vi "Automatic Teller Machine (ATM).vi"() -> ()   [LabVIEW 2016]
uses:
  Controls/State.ctl
panel:
  in  "Enter":bool
  in  "User Input":string
  in  "Right Buttons":T1
  out "Right Menu":T2
  in  "Left Buttons":T1
  out "Left Menu":T2
  in  "Card Simulator":bool
  out "ATM Messages":string
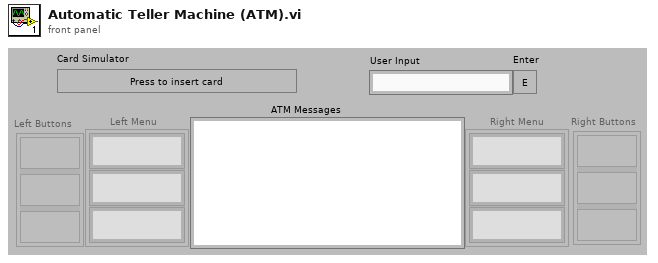
[diagram p1: front panel]
types:
  T1 = cluster{"Func Button":bool, "Func Button 2":bool, "Func Button 3":bool}
  T2 = cluster{"RFS String":string, "RFS String 2":string, "RFS String 3":string}
  T3 = typedef "State.ctl" = enum16{"Start", "Idle", "Deposit", "Withdraw", "FastCash", "None", "BalanceInquiry", "ReturnCard"}
  T4 = enum16{"CheckAccountNumber", "ReturnInfo", "Deposit", "Withdraw"}
  T5 = enum8{"Enabled", "Disabled", "Disabled and Grayed Out"}
  T6 = typedef "Account.ctl" = cluster{"Number":string, "FirstName":string, "LastName":string, "Balance":string}
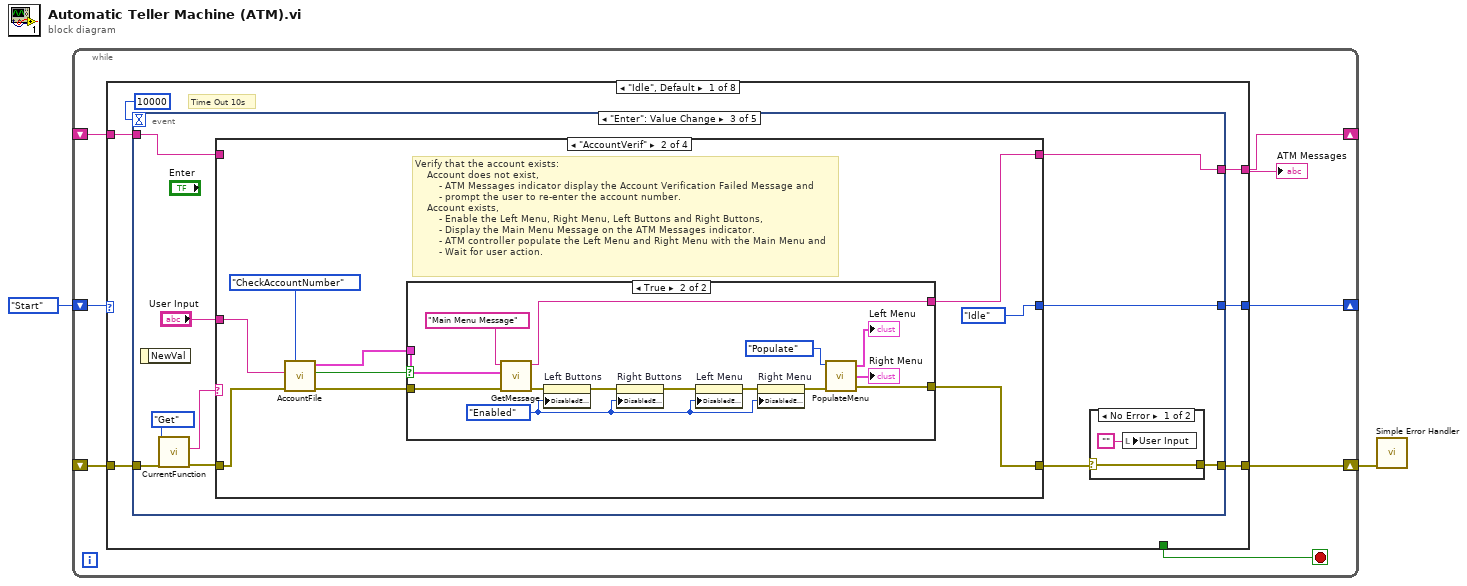
[diagram p0: block diagram]
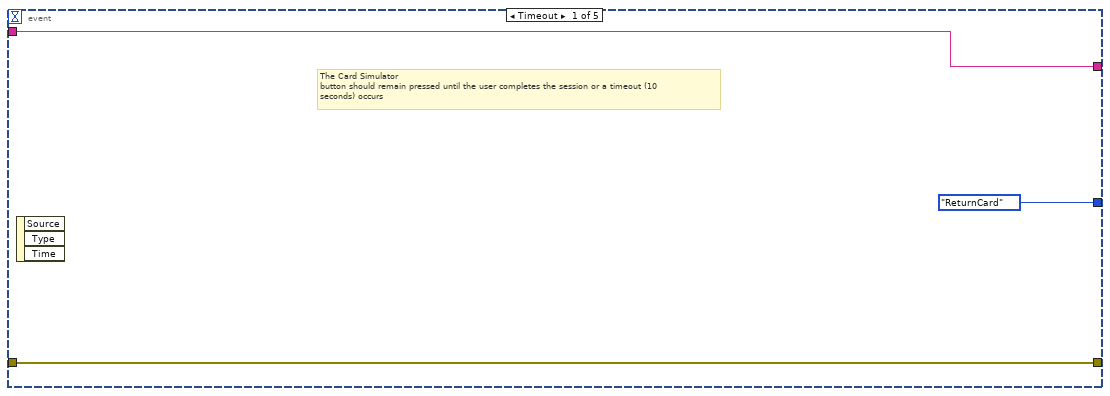
[diagram p2: hidden frame]
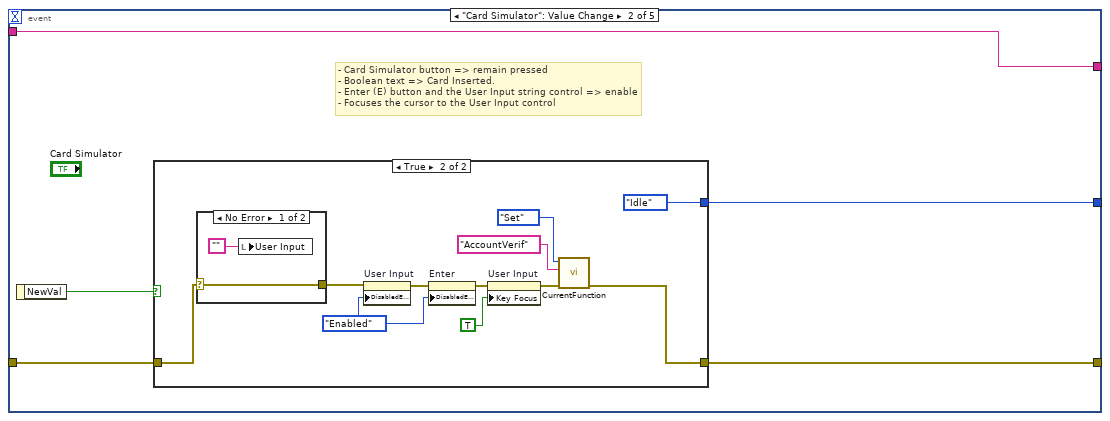
[diagram p3: hidden frame]
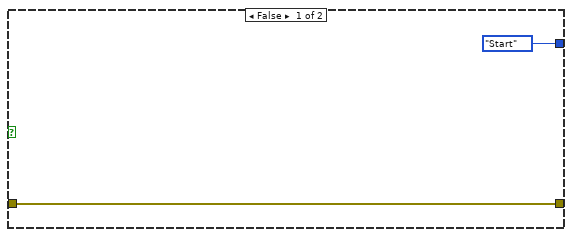
[diagram p4: hidden frame]
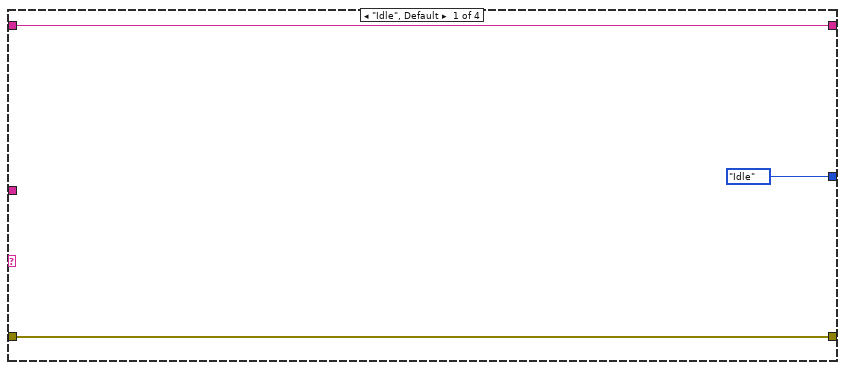
[diagram p7: hidden frame]
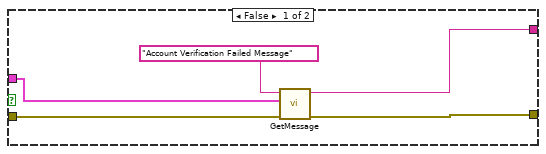
[diagram p8: hidden frame]
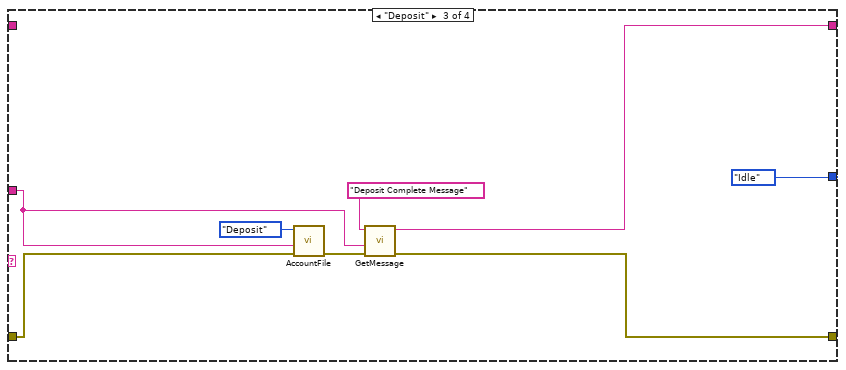
[diagram p9: hidden frame]
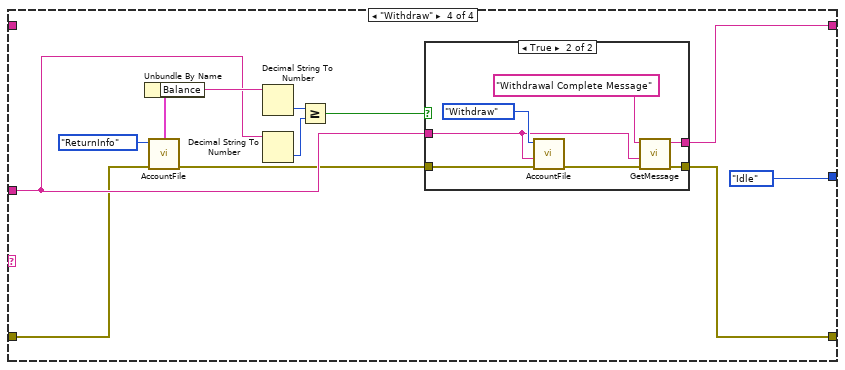
[diagram p10: hidden frame]
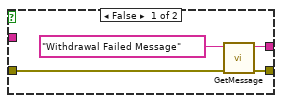
[diagram p11: hidden frame]
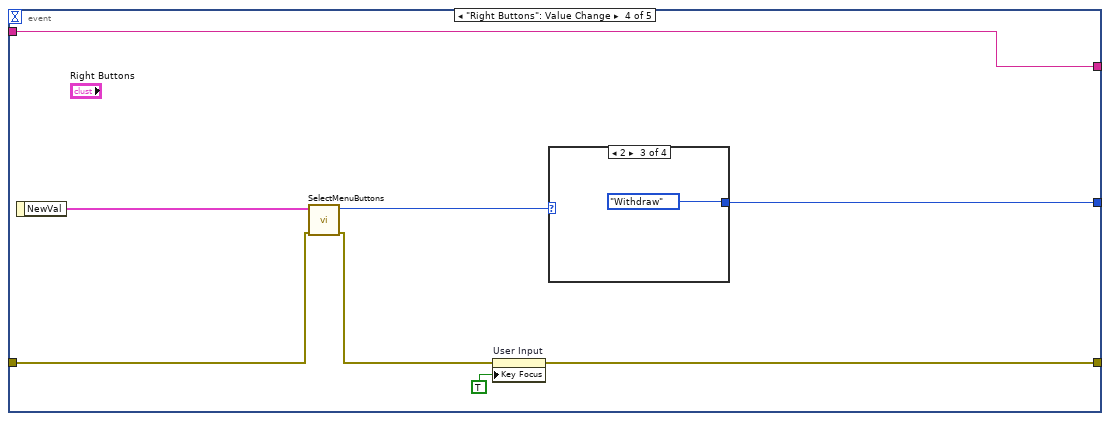
[diagram p12: hidden frame]
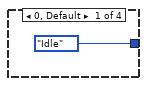
[diagram p13: hidden frame]
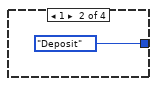
[diagram p14: hidden frame]
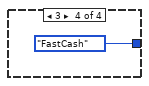
[diagram p15: hidden frame]
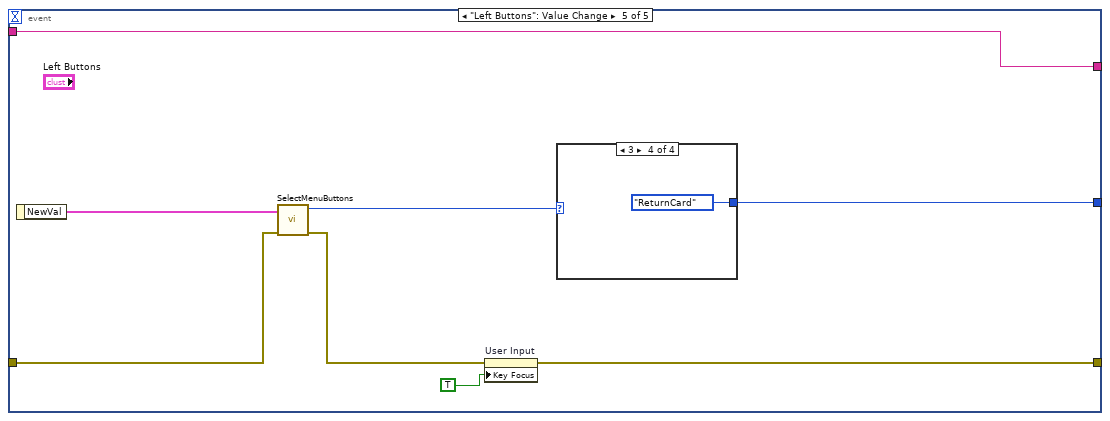
[diagram p16: hidden frame]
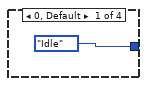
[diagram p17: hidden frame]
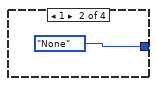
[diagram p18: hidden frame]
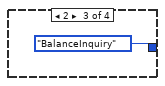
[diagram p19: hidden frame]
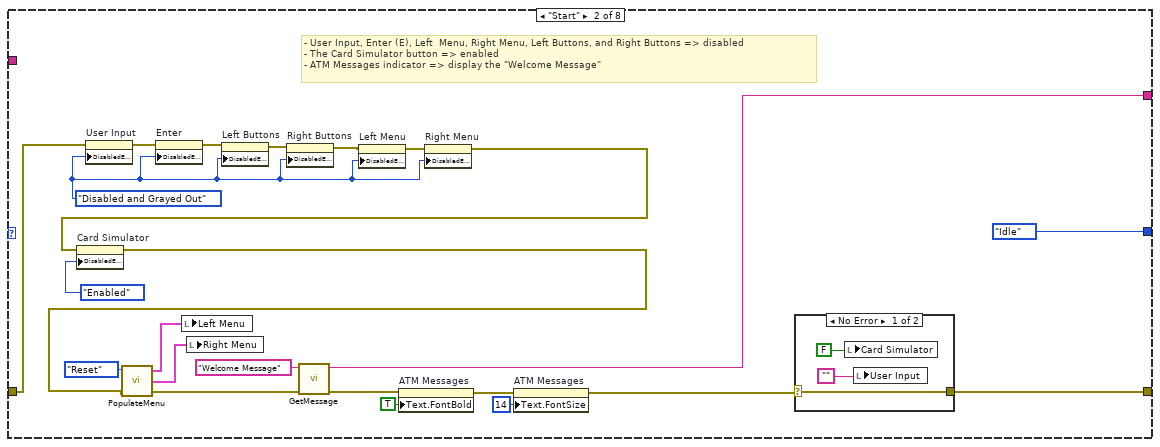
[diagram p20: hidden frame]
diagram:
  n1 = while {
    shift-right: [w3] -> _
    shift-left: State."Start" -> [w9]
    shift-right: [w8] -> w1
    shift-left: _ -> [w7]
    shift-right: [w5] -> _
    shift-left: _ -> [w4]
    stop <- w6 stop-if-true
    n2 = case shown="\"Idle\", Default" w9 {
      tunnel: [w12 State."Idle" _ State."Idle" State."Idle" State."Idle" State."Idle" State."Idle"] -> w3
      tunnel: [w13 w140 w169 w195 w207 w215 w237 w240] -> w8
      tunnel: w7 -> [w14 w139 w168 w194 w206 w214 w237 w242]
      tunnel: [_ _ TRUE _ _ _ _ _] -> w6
      tunnel: [w11 w151 w180 w197 w209 w217 "" ("Message") w243] -> w5
      tunnel: w4 -> [w10 _ _ _ _ _ _ _]
      frame "Idle", Default {
        # "Time Out 10s"
        n3 = event shown="[2] \"Enter\": Value Change" {
          selector: _ -> [_ _ _ _ _]
          dyn-events: _ -> [_ _ _ _ _]
          timeout: 10000 -> [_ _ _ _ _]
          tunnel: [State."ReturnCard" w21 w49 w120 w134] -> w12
          tunnel: w14 -> [w16 w20 w43 w116 w128]
          tunnel: [w16 w19 w40 w117 w131] -> w13
          tunnel: [w17 w23 w45 w119 w133] -> w11
          tunnel: w10 -> [w17 w23 w44 w119 w133]
          event Timeout {
            # "The Card Simulator \nbutton should remain pressed until the user completes the session or a timeout (10 \nseconds) occurs"
            n4 = event-data() -> ()  [unwired: 1 in, 3 out]
          }
          event "Card Simulator": Value Change {
            # "- Card Simulator button => remain pressed \n- Boolean text => Card Inserted. \n- Enter (E) button and the User Input string control => enable \n- Focuses the cursor to the User Input control"
            n5 = event-data() -> ("NewVal"=w22:bool)  [unwired: 1 in]
            n6 = case shown="True" w22 {
              tunnel: [State."Start" State."Idle"] -> w21
              tunnel: w20 -> [w24 w28]
              tunnel: [w24 w26] -> w19
              frame False {
              }
              frame True {
                w36 = T5."Enabled" ("Disabled")
                n7 = case shown="No Error" w28 {
                  selector: w28 -> [w37 w39]
                  tunnel: [w37 w39] -> w27
                  frame No Error {
                    n8 = local write "User Input"("") -> ()
                  }
                  frame Error {
                  }
                }
                n9 = property on="User Input" class="Str"(error in=w27, "DisabledEnum"=w36) -> (error out=w31:errorcluster)  [unwired: 1 in, 1 out]
                n10 = property on="Enter" class="Bool"(error in=w31, "DisabledEnum"=w36) -> (error out=w30:errorcluster)  [unwired: 1 in, 1 out]
                n11 = property on="User Input" class="Str"(error in=w30, "Key Focus"=TRUE) -> (error out=w29:errorcluster)  [unwired: 1 in, 1 out]
                n12 = call "CurrentFunction.vi"("error in"=w29, "Function In"="AccountVerif", "Action"=enum16{"Set", "Get"}."Set") -> ("error out"=w26:errorcluster)  [unwired: 7 in, 1 out]
              }
            }
          }
          event "Enter": Value Change {
            n13 = event-data() -> ()  [unwired: 1 in, 1 out]
            n14 = call "CurrentFunction.vi"("error in"=w43, "Action"=enum16{"Set", "Get"}."Get") -> ("error out"=w42:errorcluster, "Function Out"=w47:string)  [unwired: 8 in]
            n15 = case shown="\"AccountVerif\"" w47 {
              tunnel: w42 -> [w54 w62 w86 w94]
              tunnel: [w54 w64 w84 w92] -> w41
              tunnel: [State."Idle" State."Idle" State."Idle" State."Idle"] -> w49
              tunnel: "User Input" -> [_ w58 w88 w97]
              tunnel: [w53 w57 w87 w95] -> w45
              tunnel: w44 -> [w53 _ _ _]
              frame "Idle", Default {
              }
              frame "AccountVerif" {
                # "Verify that the account exists:\n    Account does not exist, \n        - ATM Messages indicator display the Account Verification Failed Message and \n        - prompt the user to re-enter the account number.  \n    Account exists, \n        - Enable the Left Menu, Right Menu, Left Buttons and Right Buttons, \n        - Display the Main Menu Message on the ATM Messages indicator. \n        - ATM controller populate the Left Menu and Right Menu with the Main Menu and \n        - Wait for user action."
                n16 = call "AccountFile.vi"("error in"=w62, "PIN"=w58, "Enum"=T4."CheckAccountNumber") -> ("error out"=w61:errorcluster, "Account Exist"=w56:bool, "Account"=w59:T6)  [unwired: 6 in]
                n17 = case shown="True" w56 {
                  tunnel: w61 -> [w68 w78]
                  tunnel: [w67 w75] -> w64
                  tunnel: w59 -> [w66 w73]
                  tunnel: [w65 w72] -> w57
                  frame False {
                    n18 = call "GetMessage.vi"("error in"=w68, "Account"=w66, "Message Type"="Account Verification Failed Message") -> ("error out"=w67:errorcluster, "Message"=w65:string)  [unwired: 7 in]
                  }
                  frame True {
                    w79 = T5."Enabled" ("Disabled")
                    n19 = call "GetMessage.vi"("error in"=w78, "Account"=w73, "Message Type"="Main Menu Message") -> ("error out"=w77:errorcluster, "Message"=w72:string)  [unwired: 7 in]
                    n20 = property on="Left Buttons" class="Clust"(error in=w77, "DisabledEnum"=w79) -> (error out=w82:errorcluster)  [unwired: 1 in, 1 out]
                    n21 = property on="Right Buttons" class="Clust"(error in=w82, "DisabledEnum"=w79) -> (error out=w81:errorcluster)  [unwired: 1 in, 1 out]
                    n22 = property on="Left Menu" class="Clust (strict)"(error in=w81, "DisabledEnum"=w79) -> (error out=w80:errorcluster)  [unwired: 1 in, 1 out]
                    n23 = property on="Right Menu" class="Clust (strict)"(error in=w80, "DisabledEnum"=w79) -> (error out=w76:errorcluster)  [unwired: 1 in, 1 out]
                    n24 = call "PopulateMenu.vi"("Enum"=enum16{"Reset", "Populate"}."Populate", "error in"=w76) -> ("Left Menu"=→"Left Menu":T2, "Right Menu"=→"Right Menu":T2, "error out"=w75:errorcluster)  [unwired: 4 in]
                  }
                }
              }
              frame "Deposit" {
                n25 = call "AccountFile.vi"("error in"=w86, "Amount"=w88, "Enum"=T4."Deposit") -> ("error out"=w85:errorcluster)  [unwired: 6 in, 2 out]
                n26 = call "GetMessage.vi"("error in"=w85, "Amout"=w88, "Message Type"="Deposit Complete Message") -> ("error out"=w84:errorcluster, "Message"=w87:string)  [unwired: 7 in]
              }
              frame "Withdraw" {
                n27 = call "AccountFile.vi"("error in"=w94, "Enum"=T4."ReturnInfo") -> ("error out"=w93:errorcluster, "Account"=w102:T6)  [unwired: 7 in, 1 out]
                n28 = Unbundle By Name(w102) -> ("Balance"=w101:string)
                n29 = Decimal String To Number(string=w101) -> (number=w100:i32)  [unwired: 2 in, 1 out]
                n30 = Decimal String To Number(string=w97) -> (number=w99:i32)  [unwired: 2 in, 1 out]
                n31 = Greater Or Equal?(x=w100, y=w99) -> (x >= y?=w98:bool)
                n32 = case shown="True" w98 {
                  tunnel: w97 -> [_ w112]
                  tunnel: [w106 w111] -> w95
                  tunnel: w93 -> [w105 w110]
                  tunnel: [w104 w108] -> w92
                  frame False {
                    n33 = call "GetMessage.vi"("error in"=w105, "Message Type"="Withdrawal Failed Message" ("ATM Messages")) -> ("error out"=w104:errorcluster, "Message"=w106:string)  [unwired: 8 in]
                  }
                  frame True {
                    n34 = call "AccountFile.vi"("error in"=w110, "Amount"=w112, "Enum"=T4."Withdraw") -> ("error out"=w109:errorcluster)  [unwired: 6 in, 2 out]
                    n35 = call "GetMessage.vi"("error in"=w109, "Amout"=w112, "Message Type"="Withdrawal Complete Message" ("ATM Messages")) -> ("error out"=w108:errorcluster, "Message"=w111:string)  [unwired: 7 in]
                  }
                }
              }
            }
            n36 = case shown="No Error" w41 {
              selector: w41 -> [w50 w52]
              tunnel: [w50 w52] -> w40
              frame No Error {
                n37 = local write "User Input"("") -> ()
              }
              frame Error {
              }
            }
          }
          event "Right Buttons": Value Change {
            n38 = event-data() -> ("NewVal"=w122:T1)  [unwired: 1 in]
            n39 = call "SelectMenuButtons.vi"("error in"=w116, "NewVal"=w122) -> ("error out"=w115:errorcluster, "Numeric"=w121:u32)  [unwired: 8 in]
            n40 = property on="User Input" class="Str"(error in=w115, "Key Focus"=TRUE) -> (error out=w117:errorcluster)  [unwired: 1 in, 1 out]
            n41 = case shown="2" w121 {
              tunnel: [State."Idle" State."Deposit" State."Withdraw" State."FastCash"] -> w120
              frame 0, Default {
              }
              frame 1 {
              }
              frame 2 {
              }
              frame 3 {
              }
            }
          }
          event "Left Buttons": Value Change {
            n42 = event-data() -> ("NewVal"=w130:T1)  [unwired: 1 in]
            n43 = call "SelectMenuButtons.vi"("error in"=w128, "NewVal"=w130) -> ("error out"=w127:errorcluster, "Numeric"=w129:u32)  [unwired: 8 in]
            n44 = property on="User Input" class="Str"(error in=w127, "Key Focus"=TRUE) -> (error out=w131:errorcluster)  [unwired: 1 in, 1 out]
            n45 = case shown="3" w129 {
              tunnel: [State."Idle" State."None" State."BalanceInquiry" State."ReturnCard"] -> w134
              frame 0, Default {
              }
              frame 1 {
              }
              frame 2 {
              }
              frame 3 {
              }
            }
          }
        }
      }
      frame "Start" {
        w160 = T5."Disabled and Grayed Out" ("Disabled")
        # "- User Input, Enter (E), Left  Menu, Right Menu, Left Buttons, and Right Buttons => disabled  \n- The Card Simulator button => enabled \n- ATM Messages indicator => display the \"Welcome Message\""
        n46 = property on="User Input" class="Str"(error in=w139, "DisabledEnum"=w160) -> (error out=w157:errorcluster)  [unwired: 1 in, 1 out]
        n47 = property on="Enter" class="Bool"(error in=w157, "DisabledEnum"=w160) -> (error out=w156:errorcluster)  [unwired: 1 in, 1 out]
        n48 = property on="Left Buttons" class="Clust"(error in=w156, "DisabledEnum"=w160) -> (error out=w155:errorcluster)  [unwired: 1 in, 1 out]
        n49 = property on="Right Buttons" class="Clust"(error in=w155, "DisabledEnum"=w160) -> (error out=w154:errorcluster)  [unwired: 1 in, 1 out]
        n50 = property on="Left Menu" class="Clust (strict)"(error in=w154, "DisabledEnum"=w160) -> (error out=w153:errorcluster)  [unwired: 1 in, 1 out]
        n51 = property on="Right Menu" class="Clust (strict)"(error in=w153, "DisabledEnum"=w160) -> (error out=w152:errorcluster)  [unwired: 1 in, 1 out]
        n52 = property on="Card Simulator" class="Bool (strict)"(error in=w152, "DisabledEnum"=T5."Enabled" ("Disabled")) -> (error out=w146:errorcluster)  [unwired: 1 in, 1 out]
        n53 = call "PopulateMenu.vi"("Enum"=enum16{"Reset", "Populate"}."Reset", "error in"=w146) -> ("Left Menu"=w148:T2, "Right Menu"=w147:T2, "error out"=w150:errorcluster)  [unwired: 4 in]
        n54 = local write "Left Menu"(w148) -> ()
        n55 = local write "Right Menu"(w147) -> ()
        n56 = call "GetMessage.vi"("error in"=w150, "Message Type"="Welcome Message" ("ATM Messages")) -> ("error out"=w145:errorcluster, "Message"=w151:string)  [unwired: 8 in]
        n57 = property on="ATM Messages" class="Str"(error in=w145, "Text.FontBold"=TRUE ("Text.Font:Bold")) -> (error out=w144:errorcluster)  [unwired: 1 in, 1 out]
        n58 = property on="ATM Messages" class="Str"(error in=w144, "Text.FontSize"=u32 14 ("Text.Font:Size")) -> (error out=w141:errorcluster)  [unwired: 1 in, 1 out]
        n59 = case shown="No Error" w141 {
          selector: w141 -> [w164 w165]
          tunnel: [w164 w165] -> w140
          frame No Error {
            n60 = local write "Card Simulator"(FALSE ("Card Simulator")) -> ()
            n61 = local write "User Input"("") -> ()
          }
          frame Error {
          }
        }
      }
      frame "ReturnCard" {
        w188 = T5."Disabled and Grayed Out" ("Disabled")
        n62 = property on="User Input" class="Str"(error in=w168, "DisabledEnum"=w188) -> (error out=w186:errorcluster)  [unwired: 1 in, 1 out]
        n63 = property on="Enter" class="Bool"(error in=w186, "DisabledEnum"=w188) -> (error out=w185:errorcluster)  [unwired: 1 in, 1 out]
        n64 = property on="Left Buttons" class="Clust"(error in=w185, "DisabledEnum"=w188) -> (error out=w184:errorcluster)  [unwired: 1 in, 1 out]
        n65 = property on="Right Buttons" class="Clust"(error in=w184, "DisabledEnum"=w188) -> (error out=w183:errorcluster)  [unwired: 1 in, 1 out]
        n66 = property on="Left Menu" class="Clust (strict)"(error in=w183, "DisabledEnum"=w188) -> (error out=w182:errorcluster)  [unwired: 1 in, 1 out]
        n67 = property on="Right Menu" class="Clust (strict)"(error in=w182, "DisabledEnum"=w188) -> (error out=w181:errorcluster)  [unwired: 1 in, 1 out]
        n68 = property on="Card Simulator" class="Bool (strict)"(error in=w181, "DisabledEnum"=T5."Enabled" ("Disabled")) -> (error out=w175:errorcluster)  [unwired: 1 in, 1 out]
        n69 = call "PopulateMenu.vi"("Enum"=enum16{"Reset", "Populate"}."Reset", "error in"=w175) -> ("Left Menu"=w177:T2, "Right Menu"=w176:T2, "error out"=w179:errorcluster)  [unwired: 4 in]
        n70 = local write "Left Menu"(w177) -> ()
        n71 = local write "Right Menu"(w176) -> ()
        n72 = call "GetMessage.vi"("error in"=w179, "Message Type"="Session Terminate Message" ("ATM Messages")) -> ("error out"=w174:errorcluster, "Message"=w180:string)  [unwired: 8 in]
        n73 = property on="ATM Messages" class="Str"(error in=w174, "Text.FontBold"=TRUE ("Text.Font:Bold")) -> (error out=w173:errorcluster)  [unwired: 1 in, 1 out]
        n74 = property on="ATM Messages" class="Str"(error in=w173, "Text.FontSize"=u32 14 ("Text.Font:Size")) -> (error out=w170:errorcluster)  [unwired: 1 in, 1 out]
        n75 = case shown="No Error" w170 {
          selector: w170 -> [w191 w192]
          tunnel: [w191 w192] -> w169
          frame No Error {
            n76 = local write "Card Simulator"(FALSE ("Card Simulator")) -> ()
            n77 = local write "User Input"("") -> ()
          }
          frame Error {
          }
        }
      }
      frame "Deposit" {
        n78 = case shown="No Error" w194 {
          selector: w194 -> [w204 w205]
          tunnel: [w204 w205] -> w193
          frame No Error {
            n79 = local write "User Input"("") -> ()
            n80 = property on="User Input" class="Str"("Key Focus"=TRUE) -> ()  [unwired: 2 in, 2 out]
          }
          frame Error {
          }
        }
        n81 = call "CurrentFunction.vi"("error in"=w193, "Function In"="Deposit", "Action"=enum16{"Set", "Get"}."Set") -> ("error out"=w196:errorcluster)  [unwired: 7 in, 1 out]
        n82 = call "GetMessage.vi"("error in"=w196, "Message Type"="Deposit Message" ("ATM Messages")) -> ("error out"=w195:errorcluster, "Message"=w197:string)  [unwired: 8 in]
      }
      frame "Withdraw" {
        n83 = call "CurrentFunction.vi"("error in"=w206, "Function In"="Withdraw", "Action"=enum16{"Set", "Get"}."Set") -> ("error out"=w208:errorcluster)  [unwired: 7 in, 1 out]
        n84 = call "GetMessage.vi"("error in"=w208, "Message Type"="Withdrawal Message" ("ATM Messages")) -> ("error out"=w207:errorcluster, "Message"=w209:string)  [unwired: 8 in]
      }
      frame "FastCash" {
        w218 = "50"
        # "$50 Fast Cash"
        n85 = call "AccountFile.vi"("error in"=w214, "Enum"=T4."ReturnInfo") -> ("error out"=w216:errorcluster, "Account"=w223:T6)  [unwired: 7 in, 1 out]
        n86 = Unbundle By Name(w223) -> ("Balance"=w222:string)
        n87 = Decimal String To Number(string=w222) -> (number=w220:i32)  [unwired: 2 in, 1 out]
        n88 = Decimal String To Number(string=w218) -> (number=w219:i32)  [unwired: 2 in, 1 out]
        n89 = Greater Or Equal?(x=w220, y=w219) -> (x >= y?=w221:bool)
        n90 = case shown="False" w221 {
          tunnel: [w228 w235] -> w217
          tunnel: w218 -> [_ w233]
          tunnel: w216 -> [w227 w232]
          tunnel: [w226 w230] -> w215
          frame False {
            n91 = call "GetMessage.vi"("error in"=w227, "Message Type"="Withdrawal Failed Message" ("ATM Messages")) -> ("error out"=w226:errorcluster, "Message"=w228:string)  [unwired: 8 in]
          }
          frame True {
            n92 = call "AccountFile.vi"("error in"=w232, "Amount"=w233, "Enum"=T4."Withdraw") -> ("error out"=w231:errorcluster)  [unwired: 6 in, 2 out]
            n93 = call "GetMessage.vi"("error in"=w231, "Amout"=w233, "Message Type"="Withdrawal Complete Message" ("ATM Messages")) -> ("error out"=w230:errorcluster, "Message"=w235:string)  [unwired: 7 in]
          }
        }
      }
      frame "None" {
        # "for future function"
      }
      frame "BalanceInquiry" {
        n94 = call "AccountFile.vi"("error in"=w242, "Enum"=T4."ReturnInfo") -> ("error out"=w241:errorcluster, "Account"=w245:T6)  [unwired: 7 in, 1 out]
        n95 = Unbundle By Name(w245) -> ("Balance"=w244:string)
        n96 = call "GetMessage.vi"("error in"=w241, "Amout"=w244, "Message Type"="Balance Inquiry Message" ("ATM Messages")) -> ("error out"=w240:errorcluster, "Message"=w243:string)  [unwired: 7 in]
      }
    }
    "ATM Messages" <- w5
  }
  n97 = call <vilib>:"Simple Error Handler.vi"("error in (no error)"=w1) -> ()  [unwired: 4 in, 5 out]
